vi "SwerveHeadingLock2.vi"(1 "Max Driver Translation Joystick":dbl, 3 "Driver Rotation Joystick":dbl, 6 "PID Tuning Parameters":T1={"Kp"=0.1, "Ki"=0.1, "Kd"=0.1, "N-Diff"=10, "N-Int"=20, "Int Error Window"=0.5, "Max Ouput"=1.0, "Min Output"=-1.0, "Square Derivative"=FALSE, "N-Prop"=1} {"N-Prop" min=1; "Int Error Window" min=0.0; "N-Int" min=2; "N-Diff" min=2; "Kd" min=0.0; "Ki" min=0.0; "Kp" min=0.0}, 8 "Deceleration Hysteresis (ms)":u32, 10 "Heading Lock Strafe Deadband (ft/s)":dbl, 12 "External Disables":bool) -> (14 "Controller Summary":T2(graph), 17 "Joystick Rotation":dbl, 19 "Heading Lock":bool)   [LabVIEW 2019]
doc: "This VI runs a PID controller to maintain the robot's heading while translating above a specified velocity. Dropping below the velocity threshold or manually commanding a rotation will switch off the heading lock. Assumes that all of the joystick deadbands and scalings have already been applied."
uses:
  sensors.vi
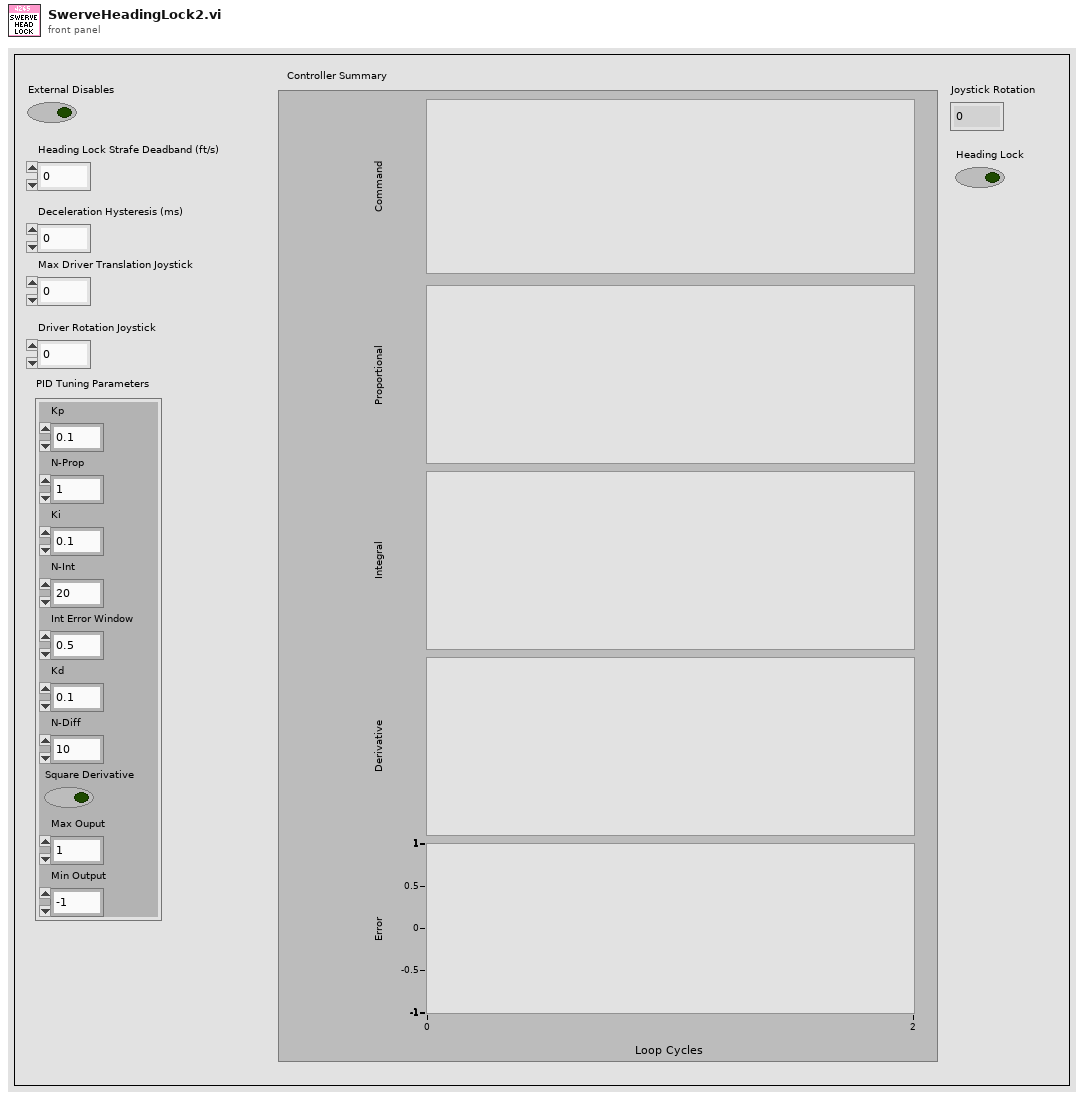
[diagram p1: front panel]
types:
  T1 = cluster{"Kp":dbl, "Ki":dbl, "Kd":dbl, "N-Diff":i32, "N-Int":i32, "Int Error Window":dbl, "Max Ouput":dbl, "Min Output":dbl, "Square Derivative":bool, "N-Prop":i32}
  T2 = cluster{"Command":dbl, "Proportional":dbl, "Integral":dbl, "Derivative":dbl, "Goal":dbl}
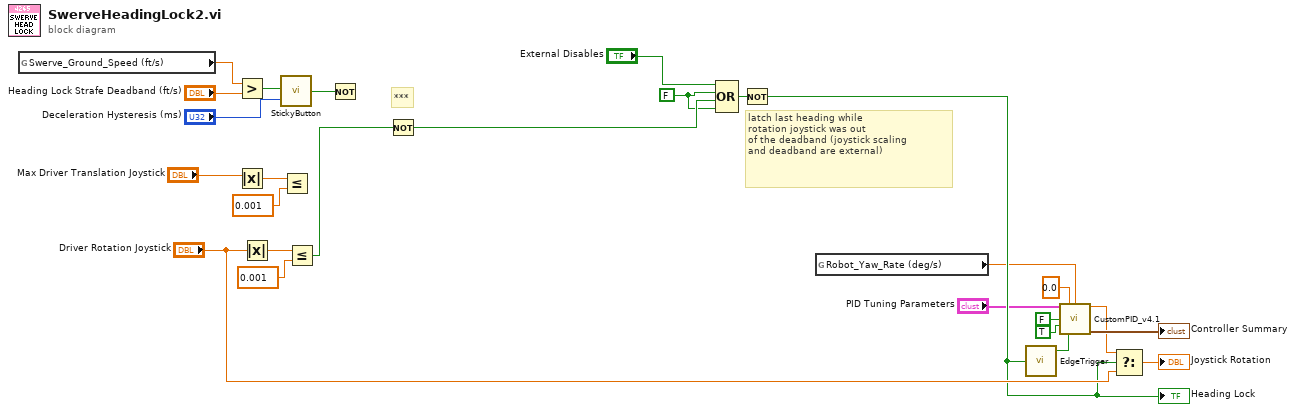
[diagram p0: block diagram]
diagram:
  w1 = FALSE ("value")
  # "***"
  # "latch last heading while\nrotation joystick was out \nof the deadband (joystick scaling \nand deadband are external)"
  n1 = global read "sensors.vi" "Swerve_Ground_Speed (ft/s)"() -> (w13:dbl)
  n2 = Greater?(x=w13, y="Heading Lock Strafe Deadband (ft/s)") -> (0:w10:bool)
  n3 = Absolute Value(x="Max Driver Translation Joystick") -> (abs(x)=w8:dbl)
  n4 = Absolute Value(x="Driver Rotation Joystick") -> (abs(x)=w23:dbl)
  n5 = call "StickyButton.vi"("Time threshold (ms)"="Deceleration Hysteresis (ms)", "Button Input"=w10) -> ("Sticky Button"=w9:bool)
  n6 = Less Or Equal?(x=w8, y=0.001) -> ()  [unwired: 1 out]
  n7 = Less Or Equal?(x=w23, y=0.001) -> (x <= y?=w12:bool)
  n8 = Not(x=w9) -> ()  [unwired: 1 out]
  n9 = Not(x=w12) -> (.not. x?=w18:bool)
  n10 = Compound Arithmetic op=OR("External Disables", w1, w18, w1) -> (w17:bool)
  n11 = Not(x=w17) -> (.not. x?=w16:bool)
  "Heading Lock" <- w16
  n12 = global read "sensors.vi" "Robot_Yaw_Rate (deg/s)"() -> (w3:dbl)
  n13 = call "EdgeTrigger.vi"("Input Signal"=w16) -> ("Rising Edge Trigger"=w24:bool)  [unwired: 2 out]
  n14 = call "CustomPID_v4.1.vi"("PID Tuning Parameters"="PID Tuning Parameters", "Goal"=0.0, "Process Variable"=w3, "Reset on Goal Change ?"=FALSE, "Use Custom Error Calculation ?"=TRUE, "Reinit"=w24) -> ("Command"=w14:dbl, "Controller Summary"=→"Controller Summary":T2)  [unwired: 6 in, 2 out]
  n15 = Select(t=w14, s=w16, f="Driver Rotation Joystick") -> (s? t:f=→"Joystick Rotation":dbl)
